vi "Query Waveform Completed (ARB Digital Modulation).vi"(8 "error in (no error)":errorcluster, 11 "VISA resource name":refnum<visa-resource-name>) -> (0 "error out":errorcluster, 2 "Completed ARB Waveform":bool, 3 "VISA resource name out":refnum<visa-resource-name>)   [LabVIEW 2018, in "Agilent PSG MXG Series.lvlib"]
doc: "Query whether the ARB waveform has completed since the last query or the last time the waveform was setup up to play. \n\n<b>Note:</b>\nIt is applicable for N5172B/82B with <b>Option 431</b> only."
uses:
  Agilent PSG MXG Series.lvlib
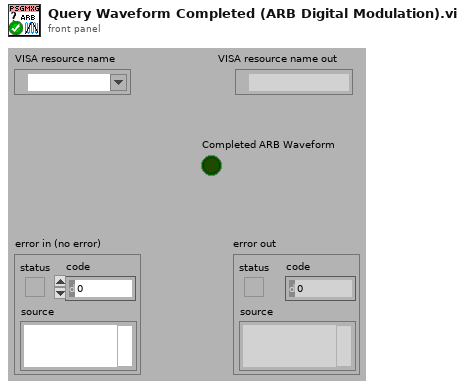
[diagram p1: front panel]
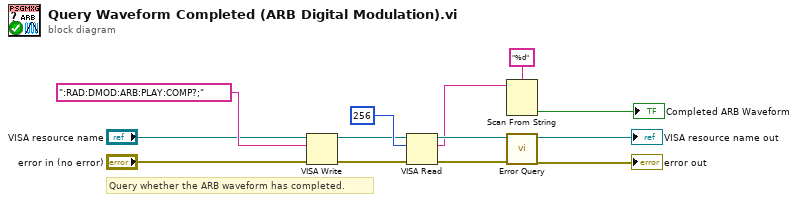
[diagram p0: block diagram]
diagram:
  # "Query whether the ARB waveform has completed."
  n1 = VISA Write(VISA resource name="VISA resource name", write buffer=":RAD:DMOD:ARB:PLAY:COMP?;", error in (no error)="error in (no error)") -> (VISA resource name out=w9:refnum<visa-resource-name>, error out=w8:errorcluster)  [unwired: 1 out]
  n2 = VISA Read(VISA resource name=w9, byte count=256, error in (no error)=w8) -> (VISA resource name out=w7:refnum<visa-resource-name>, read buffer=w1:string, error out=w6:errorcluster)  [unwired: 1 out]
  n3 = Scan From String(format string="%d", input string=w1) -> (output 1=→"Completed ARB Waveform":bool)  [unwired: 3 in, 3 out]
  n4 = call "Error Query.vi"("error in (no error)"=w6, "VISA resource name"=w7) -> ("error out"=→"error out":errorcluster, "VISA resource name out"=→"VISA resource name out":refnum<visa-resource-name>)  [unwired: 6 in, 2 out]
